vi "MatrixB_Vg_dep.vi"(0 "Vg-table String":string, 3 "Time Stamp":timestamp, 6 "Play Button":bool, 7 "Custom Folder":string, 8 "Settings":T2={"Ring 3"=1, "Ring 2"=4, "Fixed Current mkA"=0.5, "If yes, the current is:"=enum."Radio Selection 1", "Ressitance measurements?"=TRUE, "Commute DC current?"=FALSE} {"Ring 3" items=["1 kOhm", "10 kOhm", "100 kOhm", "1 Mohm", "10 mOhm"]; "Ring 2" items=["1 kOhm", "10 kOhm", "100 kOhm", "1 Mohm", "10 MOhm"]}, 9 "Instruments":T3={"Oscillator"=TRUE, "Addr 1 lock-in"=TRUE, "Addr 1 lock-in oop"=TRUE, "Addr 2 lock-in"=TRUE, "Addr 2 lock-in oop"=TRUE, "Addr 3 lock-in"=FALSE, "Addr 3 lock-in oop"=FALSE, "Voltage (Vk1)"=FALSE, "Current (Ik1)"=TRUE, "Voltage (Vk2)"=FALSE, "Current (Ik2)"=FALSE, "Voltage (Vk3)"=FALSE, "Current (Ik3)"=FALSE, "Channel 1 (Vnano1)  "=FALSE, "Channel 2 (Vnano1b)"=FALSE, "Channel 1 (Vnano2)   "=FALSE, "Channel 2 (Vnano2b)"=FALSE, "Thermometer 1 (T1)"=TRUE, "Magnetic Field (B)"=TRUE, "Capacitance (C) and Loss (L)"=FALSE}, 10 "BCluster":T4={"B1 (V)"=-1.0, "B2 (V)"=1.0, "Sweep rate, T/min"=0.5, "Time btw \npoints, sec"=1.0, "No-record rate, T/min"=0.5, "Full sweep?"=FALSE, "Odd confgurations"=TRUE} {"No-record rate, T/min" min=0.0 max=1.0 step=0.01 format="%_4f"; "B2 (V)" min=-4.0 max=4.0 step=0.1 format="%.2f"; "Time btw \npoints, sec" format="%.2f"; "Sweep rate, T/min" min=0.0 max=1.0 step=0.01 format="%_4f"; "B1 (V)" min=-4.0 max=4.0 step=0.1 format="%.2f"}, 11 "VgCluster":T1={"Starting Vg (V)"=-1.0, "Final Vg (V)"=1.0, "Step (V)"=1.0} {"Final Vg (V)" min=-4.0 max=4.0 step=0.1 format="%.2f"; "Step (V)" min=0.0 max=1.0 step=0.01 format="%_4f"; "Starting Vg (V)" min=-4.0 max=4.0 step=0.1 format="%.2f"}) -> ()   [LabVIEW 2017]
uses:
  <vilib>/Utility/file.llb/Read From Spreadsheet File (DBL).vi
panel:
  in  "No record Vg rate (V/min)":dbl=150.0
  out "Communication":string
  out "Vg Array":dbl[](array[numeric])
  out "Experiment ends at:":string
  out "Hours":dbl format="%.1f"
  out "Estimated time of experiment:":i16
  out "ArraySens":i8[](array[numeric])
  out "ArrayOsc":dbl[](array[numeric])
  out "# of configurations":i8
  out "Large Array":bool[][][](array[boolean])
  out "Contact configuration file (*.conf)":path
  # "1"
  # "hours"
  # "min.="
  # "Values of Vg can be also entered as the table by copying\nand pasting a column of numbers in a \"Vg table\" string at the \nfar right side of this window."
  # "Lock-in Amplifiers"
  # "Temperature"
  # "SourceMeters"
  # "Nanovoltmeters"
  # "Main"
  # "(not recommended, too slow)"
  # "Magnetic Field"
  # "Capacitance & Loss"
  # "(not recommended, too slow)"
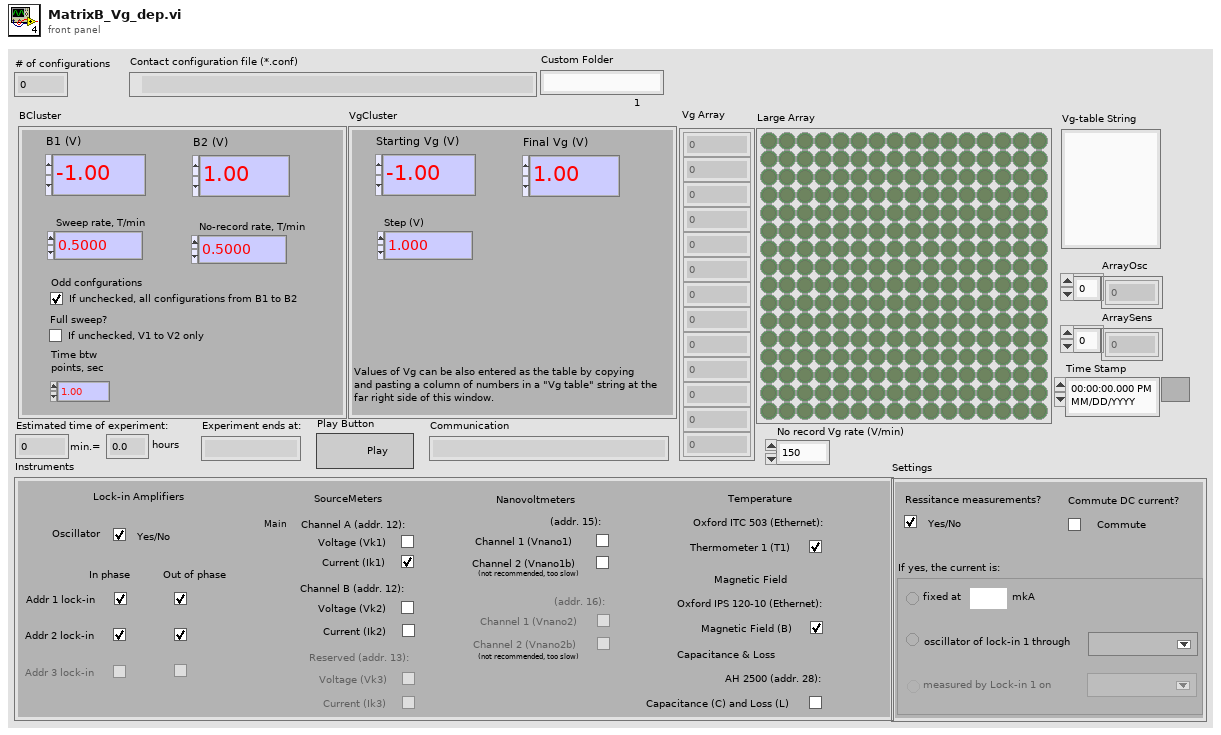
[diagram p1: front panel]
types:
  T1 = cluster{"Starting Vg (V)":dbl, "Final Vg (V)":dbl, "Step (V)":dbl}
  T2 = cluster{"Ring 3":u16, "Ring 2":u16, "Fixed Current mkA":dbl, "If yes, the current is:":enum32{"Radio Selection 1", "Radio Selection 2", "Radio Selection 3"}, "Ressitance measurements?":bool, "Commute DC current?":bool}
  T3 = cluster{"Oscillator":bool, "Addr 1 lock-in":bool, "Addr 1 lock-in oop":bool, "Addr 2 lock-in":bool, "Addr 2 lock-in oop":bool, "Addr 3 lock-in":bool, "Addr 3 lock-in oop":bool, "Voltage (Vk1)":bool, "Current (Ik1)":bool, "Voltage (Vk2)":bool, "Current (Ik2)":bool, "Voltage (Vk3)":bool, "Current (Ik3)":bool, "Channel 1 (Vnano1)  ":bool, "Channel 2 (Vnano1b)":bool, "Channel 1 (Vnano2)   ":bool, "Channel 2 (Vnano2b)":bool, "Thermometer 1 (T1)":bool, "Magnetic Field (B)":bool, "Capacitance (C) and Loss (L)":bool}
  T4 = cluster{"B1 (V)":dbl, "B2 (V)":dbl, "Sweep rate, T/min":dbl, "Time btw \npoints, sec":dbl, "No-record rate, T/min":dbl, "Full sweep?":bool, "Odd confgurations":bool}
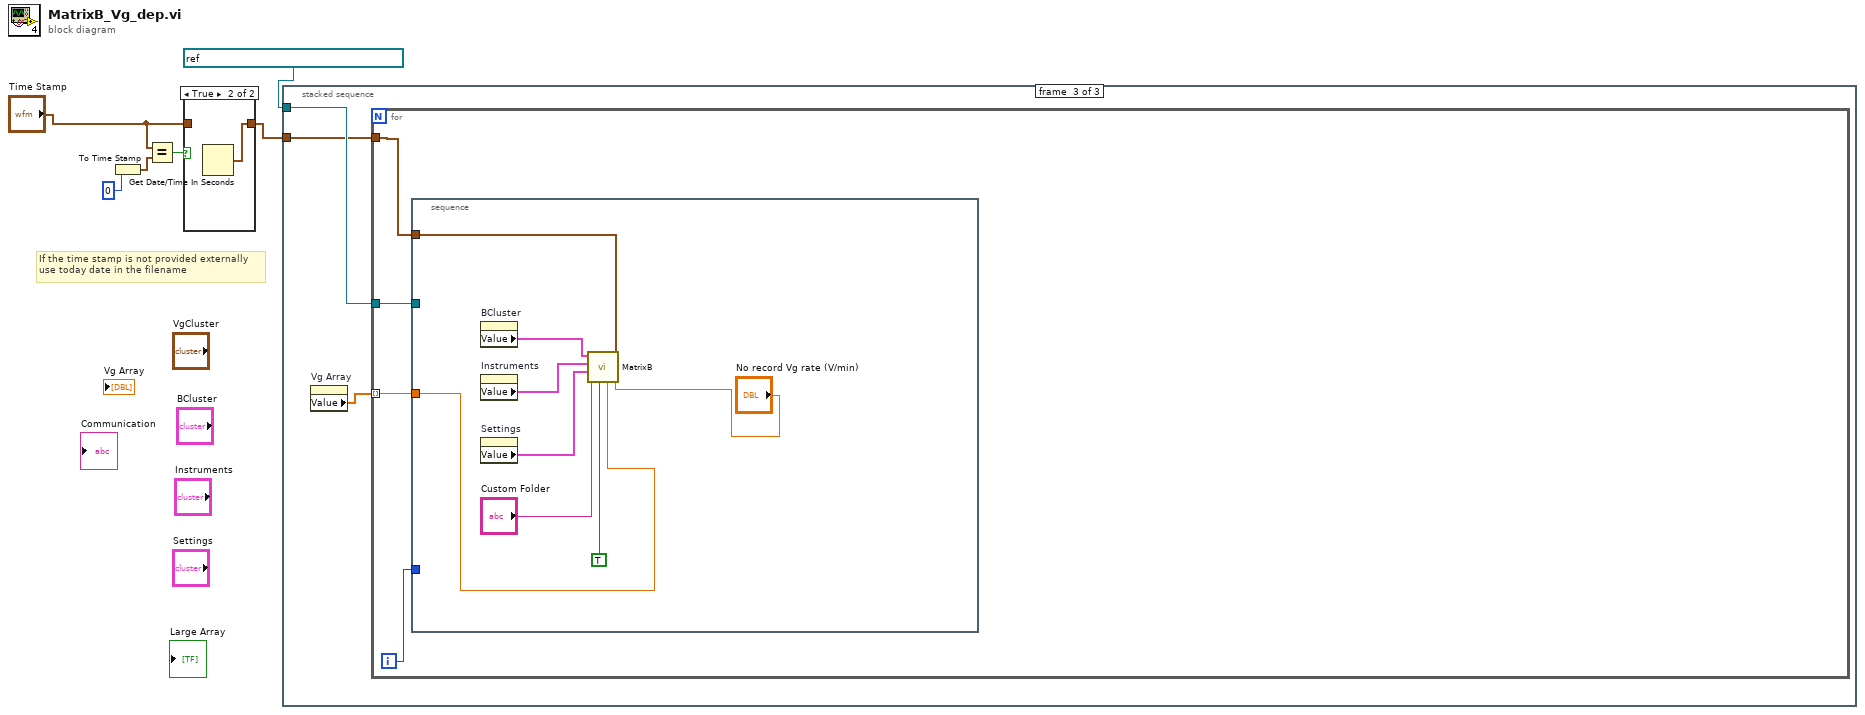
[diagram p0: block diagram]
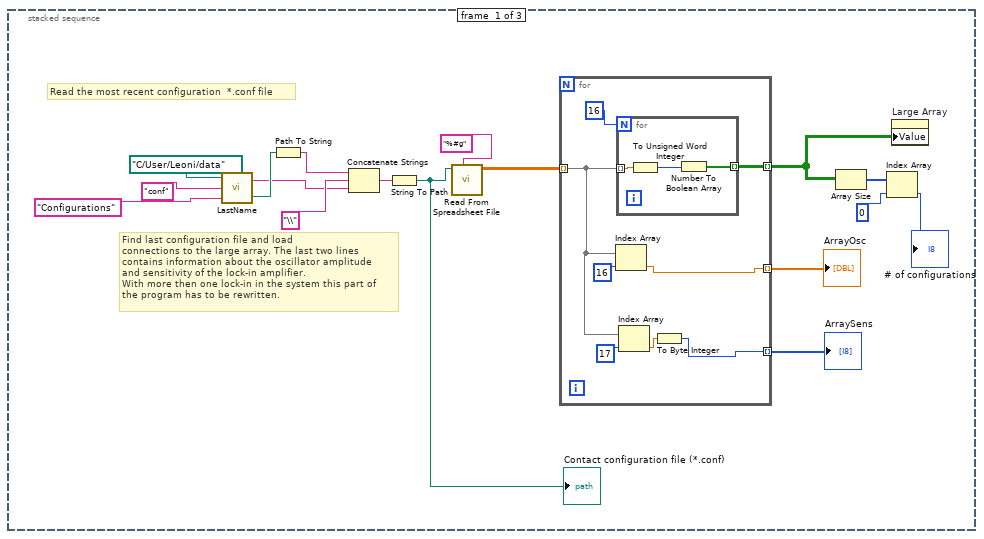
[diagram p3: hidden frame]
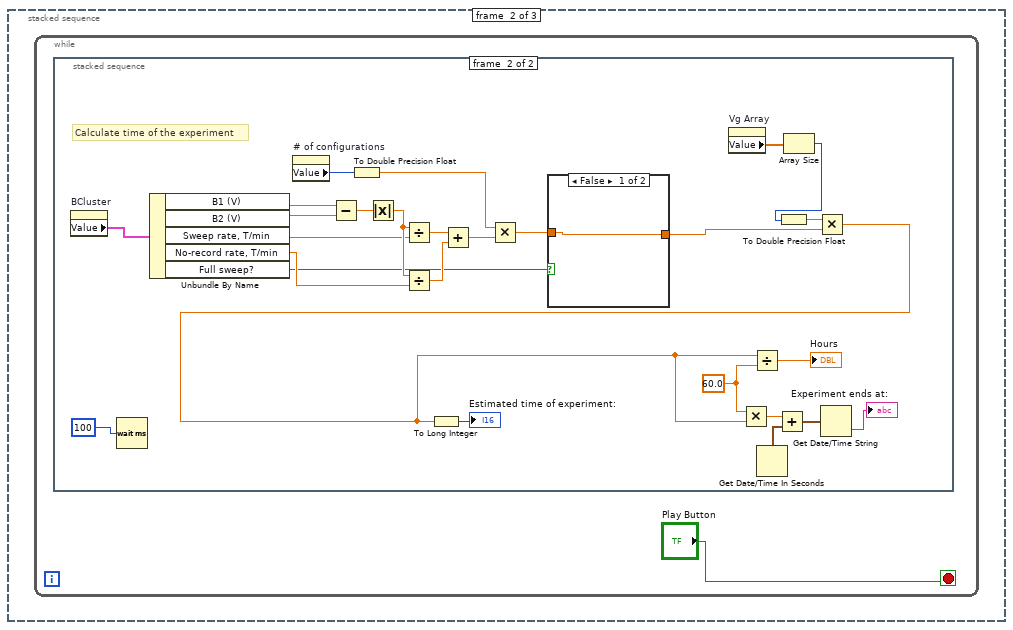
[diagram p4: hidden frame]
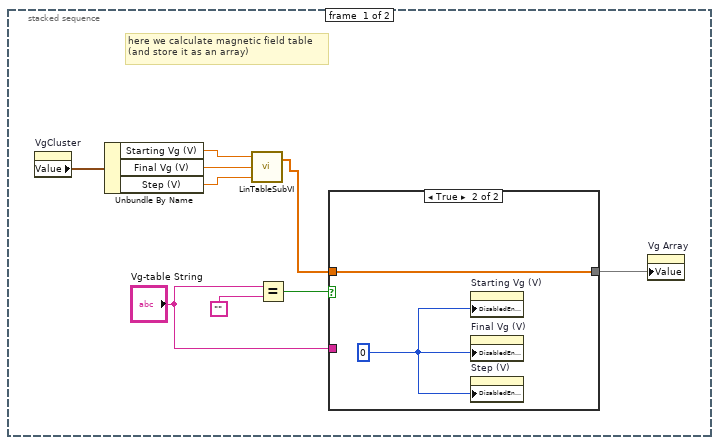
[diagram p5: hidden frame]
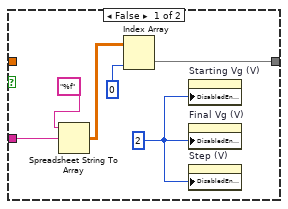
[diagram p6: hidden frame]
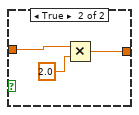
[diagram p7: hidden frame]
diagram:
  # "If the time stamp is not provided externally\nuse today date in the filename"
  n1 = To Time Stamp(1:0) -> (0:w5:timestamp)
  n2 = Equal?(x="Time Stamp", y=w5) -> (x = y?=w4:bool)
  n3 = case shown="True" w4 {
    tunnel: "Time Stamp" -> [w7 _]
    tunnel: [w7 w8] -> w2
    frame False {
    }
    frame True {
      n4 = Get Date/Time In Seconds() -> (seconds since 1Jan1904=w8:timestamp)
    }
  }
  n5 = stacked-sequence {
    tunnel: w2 -> [_ _ w86]
    tunnel: refnum<visa-resource-name> "TCPIP0::192.168.128.2::7020::SOCKET" ("VISA resource name") -> [_ _ w88]
    frame #0 {
      # "Read the most recent configuration  *.conf file"
      # "Find last configuration file and load \nconnections to the large array. The last two lines \ncontains information about the oscillator amplitude\nand sensitivity of the lock-in amplifier.\nWith more then one lock-in in the system this part of \nthe program has to be rewritten."
      n6 = call "LastName.vi"("Custom Folder"="Configurations", "Extention"="conf", "User Data Folder"=path "C:/User/Leoni/data") -> ("created path"=w21:path, "String"=w20:string)
      n7 = Path To String(path=w21) -> (string=w25:string)
      n8 = Concatenate Strings(w25, "\\", w20) -> (w23:string)
      n9 = String To Path(string=w23) -> (path=w11:path)
      "Contact configuration file (*.conf)" <- w11
      n10 = call-poly <vilib>:"Read From Spreadsheet File.vi"("format (%.3f)"="%#g", "file path (dialog if empty)"=w11) -> ("all rows"=w16:dbl[][])  [unwired: 5 in, 4 out]
      n11 = for {
        tunnel: w16 -> [w29] mode=indexing
        tunnel: [w33] -> w13 mode=indexing
        tunnel: [w28] -> w10 mode=indexing
        tunnel: [w27] -> w9 mode=indexing
        n12 = Index Array(array=w29, index=16) -> (element=w28:dbl)
        n13 = for {
          N: 16 -> [_]
          tunnel: w29 -> [w36] mode=indexing
          tunnel: [w34] -> w33 mode=indexing
          n14 = To Unsigned Word Integer(number=w36) -> (unsigned 16bit integer=w35:u16)
          n15 = Number To Boolean Array(number=w35) -> (Boolean array=w34:bool[])
        }
        n16 = Index Array(array=w29, index=17) -> (element=w30:dbl)
        n17 = To Byte Integer(number=w30) -> (8bit integer=w27:i8)
      }
      "ArrayOsc" <- w10
      "ArraySens" <- w9
      n18 = Array Size(array=w13) -> (size(s)=w15:i32[])
      n19 = Index Array(array=w15, index=0) -> (element=→"# of configurations":i32)
      n20 = property on="Large Array" class="Arr (strict)"("Value"=w13) -> ()  [unwired: 2 in, 2 out]
    }
    frame #1 {
      n21 = while {
        stop <- "Play Button" stop-if-true
        n22 = stacked-sequence {
          frame #0 {
            # "here we calculate magnetic field table\n(and store it as an array)"
            n23 = property on="VgCluster" class="Clust (strict)"() -> ("Value"=w42:T1)  [unwired: 2 in, 2 out]
            n24 = Unbundle By Name(w42) -> ("Starting Vg (V)"=w41:dbl, "Final Vg (V)"=w40:dbl, "Step (V)"=w39:dbl)
            n25 = call "LinTableSubVI.vi"("Step"=w39, "Final"=w40, "Initial"=w41) -> ("Array"=w46:dbl[])  [unwired: 1 in]
            n26 = Equal?(x="Vg-table String", y="") -> (x = y?=w43:bool)
            n27 = case shown="True" w43 {
              tunnel: [w49 w54] -> w38
              tunnel: w46 -> [_ w54]
              tunnel: "Vg-table String" -> [w48 _]
              frame False {
                w47 = 2
                n28 = Spreadsheet String To Array(format string="%f", spreadsheet string=w48) -> (array=w51:dbl[][])  [unwired: 2 in]
                n29 = Index Array(array=w51, index (col)=0) -> (element=w49:dbl[])  [unwired: 1 in]
                n30 = property on="Starting Vg (V)" class="DigNum (strict)"("DisabledEnum"=w47) -> ()  [unwired: 2 in, 2 out]
                n31 = property on="Final Vg (V)" class="DigNum (strict)"("DisabledEnum"=w47) -> ()  [unwired: 2 in, 2 out]
                n32 = property on="Step (V)" class="DigNum (strict)"("DisabledEnum"=w47) -> ()  [unwired: 2 in, 2 out]
              }
              frame True {
                w53 = 0
                n33 = property on="Starting Vg (V)" class="DigNum (strict)"("DisabledEnum"=w53) -> ()  [unwired: 2 in, 2 out]
                n34 = property on="Final Vg (V)" class="DigNum (strict)"("DisabledEnum"=w53) -> ()  [unwired: 2 in, 2 out]
                n35 = property on="Step (V)" class="DigNum (strict)"("DisabledEnum"=w53) -> ()  [unwired: 2 in, 2 out]
              }
            }
            n36 = property on="Vg Array" class="Arr (strict)"("Value"=w38) -> ()  [unwired: 2 in, 2 out]
          }
          frame #1 {
            w61 = 60.0
            # "Calculate time of the experiment"
            n37 = property on="BCluster" class="Clust (strict)"() -> ("Value"=w80:T4)  [unwired: 2 in, 2 out]
            n38 = Wait (ms)(milliseconds to wait=100) -> ()  [unwired: 1 out]
            n39 = Unbundle By Name(w80) -> ("B1 (V)"=w79:dbl, "B2 (V)"=w78:dbl, "Sweep rate, T/min"=w75:dbl, "No-record rate, T/min"=w74:dbl, "Full sweep?"=w68:bool)
            n40 = property on="# of configurations" class="DigNum (strict)"() -> ("Value"=w70:i8)  [unwired: 2 in, 2 out]
            n41 = Subtract(x=w79, y=w78) -> (x-y=w77:dbl)
            n42 = To Double Precision Float(number=w70) -> (double precision float=w69:dbl)
            n43 = Absolute Value(x=w77) -> (abs(x)=w76:dbl)
            n44 = Divide(x=w76, y=w75) -> (x/y=w73:dbl)
            n45 = Divide(x=w76, y=w74) -> (x/y=w72:dbl)
            n46 = Add(x=w73, y=w72) -> (x+y=w71:dbl)
            n47 = Multiply(x=w69, y=w71) -> (x*y=w67:dbl)
            n48 = case shown="False" w68 {
              tunnel: w67 -> [w82 w85]
              tunnel: [w82 w83] -> w55
              frame False {
              }
              frame True {
                n49 = Multiply(x=w85, y=2.0) -> (x*y=w83:dbl)
              }
            }
            n50 = property on="Vg Array" class="Arr (strict)"() -> ("Value"=w59:dbl[])  [unwired: 2 in, 2 out]
            n51 = Get Date/Time In Seconds() -> (seconds since 1Jan1904=w65:timestamp)
            n52 = Array Size(array=w59) -> (size(s)=w57:i32)
            n53 = To Double Precision Float(number=w57) -> (double precision float=w58:dbl)
            n54 = Multiply(x=w58, y=w55) -> (x*y=w56:dbl)
            n55 = To Long Integer(number=w56) -> (32bit integer=→"Estimated time of experiment:":i32)
            n56 = Multiply(x=w61, y=w56) -> (x*y=w60:dbl)
            n57 = Divide(x=w56, y=w61) -> (x/y=→"Hours":dbl)
            n58 = Add(x=w60, y=w65) -> (x+y=w64:timestamp)
            n59 = Get Date/Time String(seconds (now)=w64) -> (time string=→"Experiment ends at:":string)  [unwired: 2 in, 1 out]
          }
        }
      }
    }
    frame #2 {
      n60 = property on="Vg Array" class="Arr (strict)"() -> ("Value"=w87:dbl[])  [unwired: 2 in, 2 out]
      n61 = for {
        tunnel: w88 -> [w92]
        tunnel: w87 -> [w91] mode=indexing
        tunnel: w86 -> [w89]
        i -> [w90]
        n62 = stacked-sequence {
          tunnel: w92 -> [_]
          tunnel: w91 -> [w93]
          tunnel: w90 -> [_]
          tunnel: w89 -> [w94]
          frame #0 {
            n63 = property on="BCluster" class="Clust (strict)"() -> ("Value"=w99:T4)  [unwired: 2 in, 2 out]
            n64 = property on="Instruments" class="Clust (strict)"() -> ("Value"=w95:T3)  [unwired: 2 in, 2 out]
            n65 = property on="Settings" class="Clust (strict)"() -> ("Value"=w96:T2)  [unwired: 2 in, 2 out]
            n66 = call "MatrixB.vi"("No record Vg rate (V/min)"="No record Vg rate (V/min)", "Time Stamp"=w94, "Voltage (sourse)"=w93, "Play Button"=TRUE, "Custom Folder"="Custom Folder", "Settings"=w96, "Instruments"=w95, "BCluster"=w99) -> ()  [unwired: 4 in]
          }
        }
      }
    }
  }
